vi "Filter out strings.vi"(10 "Filter out if containing this string":string, 11 "array w/ subset deleted in":string[](array[string])) -> (3 "array w/ subset deleted out":string[](array[string]))   [LabVIEW 2017]
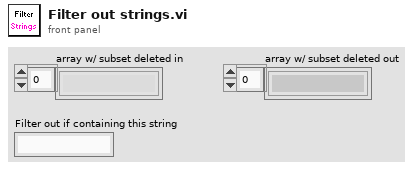
[diagram p1: front panel]
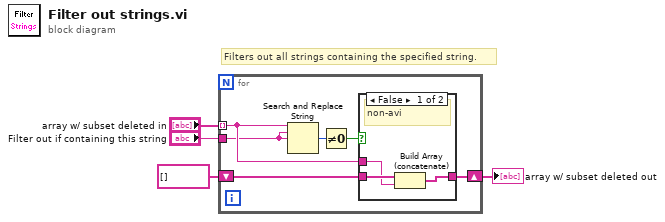
[diagram p0: block diagram]
diagram:
  # "Filters out all strings containing the specified string."
  n1 = for {
    tunnel: "array w/ subset deleted in" -> [w7] mode=indexing
    shift-right: [w6] -> w3
    shift-left: string[] [] ("array w/ subset deleted") -> [w8]
    tunnel: "Filter out if containing this string" -> [w5]
    n2 = Search and Replace String(input string=w7, search string=w5, replace string=w5) -> (number of replacements=w10:i32)  [unwired: 5 in, 3 out]
    n3 = Not Equal To 0?(x=w10) -> (x != 0?=w9:bool)
    n4 = case shown="False" w9 {
      tunnel: w8 -> [w13 w14]
      tunnel: w7 -> [w12 _]
      tunnel: [w11 w14] -> w6
      frame False {
        # "non-avi"
        n5 = Build Array (concatenate)(w13, w12) -> (w11:string[])
      }
      frame True {
        # "AVI file"
      }
    }
  }
  "array w/ subset deleted out" <- w3
